vi "Logger.Variant.FindData4.vi"() -> ()   [LabVIEW 2016] (continued)
 "D:/Maszup/WABCO/SVN/LaserMarkingStation/SOFTWARE/logs/results1/old/170419233635 899 053 814 4.tdms", "Serials"=["480003047015824401617", "480003047015824411617", "480003047015824421617", "480003047015824431617", "480003047015824441617", "480003047015824451617", "480003047015824461617", "480003047015824471617", "480003047015824481617", "480003047015824491617", "480003047015824501617", "480003047015824511617", "480003047015824521617", "480003047015824531617", "480003047015824541617", "480003047015824551617", "480003047015824561617", "480003047015824571617", "480003047015824581617", "480003047015824591617", "480003047015824601617", "480003047015824611617", "480003047015824621617", "480003047015824631617", "480003047015824641617", "480003047015824651617", "480003047015824661617", "480003047015824671617", "480003047015824681617", "480003047015824691617", "480003047015824701617", "480003047015824711617", "480003047015824721617", "480003047015824731617", "480003047015824741617", "480003047015824751617", "480003047015824761617", "480003047015824771617", "480003047015824781617", "480003047015824791617"]}, {"Product"="9650010550", "Plate"="8990538144", "Path"=path "D:/Maszup/WABCO/SVN/LaserMarkingStation/SOFTWARE/logs/results1/old/170419234304 899 053 814 4.tdms", "Serials"=["965001055001223591617", "965001055001223601617", "965001055001223611617", "965001055001223621617", "965001055001223631617", "965001055001223641617", "965001055001223651617", "965001055001223661617", "965001055001223671617", "965001055001223681617", "965001055001223691617", "965001055001223701617"]}, {"Product"="9650010550", "Plate"="8990538144", "Path"=path "D:/Maszup/WABCO/SVN/LaserMarkingStation/SOFTWARE/logs/results1/old/170419234627 899 053 814 4.tdms", "Serials"=["965001055001223711617", "965001055001223721617", "965001055001223731617", "965001055001223741617", "965001055001223761617", "965001055001223771617", "965001055001223781617", "965001055001223791617", "965001055001223801617", "965001055001223811617", "965001055001223821617"]}, {"Product"="9650010550", "Plate"="8990538144", "Path"=path "D:/Maszup/WABCO/SVN/LaserMarkingStation/SOFTWARE/logs/results1/old/170419235443 899 053 814 4.tdms", "Serials"=["965001055001223711617", "965001055001223721617"]}, {"Product"="9650010550", "Plate"="8990538144", "Path"=path "D:/Maszup/WABCO/SVN/LaserMarkingStation/SOFTWARE/logs/results1/old/170420000204 899 053 814 4.tdms", "Serials"=["965001055001223711617", "965001055001223721617", "965001055001223731617", "965001055001223741617", "965001055001223751617", "965001055001223761617", "965001055001223771617", "965001055001223781617", "965001055001223791617", "965001055001223801617", "965001055001223811617", "965001055001223821617"]}, {"Product"="9650010550", "Plate"="8990538144", "Path"=path "D:/Maszup/WABCO/SVN/LaserMarkingStation/SOFTWARE/logs/results1/old/170420000541 899 053 814 4.tdms", "Serials"=["965001055001223831617", "965001055001223841617", "965001055001223851617", "965001055001223861617", "965001055001223871617", "965001055001223881617", "965001055001223891617", "965001055001223901617", "965001055001223911617", "965001055001223921617", "965001055001223931617", "965001055001223941617"]}, {"Product"="4728901130", "Plate"="8990501474", "Path"=path "D:/Maszup/WABCO/SVN/LaserMarkingStation/SOFTWARE/logs/results1/old/170420001243 899 050 147 4.tdms", "Serials"=["472890113015857521617", "472890113015857531617", "472890113015857541617", "472890113015857551617", "472890113015857561617", "472890113015857571617", "472890113015857581617", "472890113015857591617", "472890113015857601617", "472890113015857611617", "472890113015857621617"]}, {"Product"="4728901130", "Plate"="8990501474", "Path"=path "D:/Maszup/WABCO/SVN/LaserMarkingStation/SOFTWARE/logs/results1/old/170420001628 899 050 147 4.tdms", "Serials"=["472890113015857631617", "472890113015857641617", "472890113015857651617", "472890113015857661617", "472890113015857671617", "472890113015857681617"]}, {"Product"="4728901130", "Plate"="8990501474", "Path"=path "D:/Maszup/WABCO/SVN/LaserMarkingStation/SOFTWARE/logs/results1/old/170420002155 899 050 147 4.tdms", "Serials"=["472890113015857691617", "472890113015857701617", "472890113015857711617", "472890113015857721617", "472890113015857731617", "472890113015857741617", "472890113015857751617", "472890113015857761617", "472890113015857771617", "472890113015857781617", "472890113015857791617", "472890113015857801617", "472890113015857811617", "472890113015857821617", "472890113015857831617", "472890113015857841617", "472890113015857851617", "472890113015857861617", "472890113015857871617", "472890113015857881617", "472890113015857891617", "472890113015857901617", "472890113015857911617", "472890113015857921617", "472890113015857931617", "472890113015857941617", "472890113015857951617", "472890113015857961617", "472890113015857971617", "472890113015857981617", "472890113015857991617", "472890113015858001617", "472890113015858011617", "472890113015858021617", "472890113015858031617", "472890113015858041617"]}, {"Product"="9650010550", "Plate"="8990538144", "Path"=path "D:/Maszup/WABCO/SVN/LaserMarkingStation/SOFTWARE/logs/results1/old/170420002831 899 053 814 4.tdms", "Serials"=["965001055001223711617"]}, {"Product"="4728900500", "Plate"="8990538144", "Path"=path "D:/Maszup/WABCO/SVN/LaserMarkingStation/SOFTWARE/logs/results1/old/170420004617 899 053 814 4.tdms", "Serials"=["472890050016182201617", "472890050016182211617", "472890050016182221617", "472890050016182231617", "472890050016182241617", "472890050016182251617", "472890050016182261617", "472890050016182271617", "472890050016182281617", "472890050016182291617", "472890050016182301617", "472890050016182311617", "472890050016182321617", "472890050016182331617", "472890050016182341617", "472890050016182351617", "472890050016182361617", "472890050016182371617", "472890050016182381617", "472890050016182391617", "472890050016182401617", "472890050016182411617", "472890050016182421617", "472890050016182431617", "472890050016182441617", "472890050016182451617", "472890050016182461617", "472890050016182471617", "472890050016182481617", "472890050016182491617"]}, {"Product"="4728900500", "Plate"="8990538144", "Path"=path "D:/Maszup/WABCO/SVN/LaserMarkingStation/SOFTWARE/logs/results1/old/170420005019 899 053 814 4.tdms", "Serials"=["472890050016182501617", "472890050016182511617", "472890050016182521617", "472890050016182531617", "472890050016182541617", "472890050016182551617", "472890050016182561617", "472890050016182571617", "472890050016182581617", "472890050016182591617", "472890050016182601617", "472890050016182611617", "472890050016182621617", "472890050016182631617", "472890050016182641617", "472890050016182651617", "472890050016182661617", "472890050016182671617", "472890050016182681617", "472890050016182691617", "472890050016182701617", "472890050016182711617", "472890050016182721617", "472890050016182731617", "472890050016182741617", "472890050016182751617", "472890050016182761617", "472890050016182771617", "472890050016182781617", "472890050016182791617"]}, {"Product"="4728900500", "Plate"="8990538144", "Path"=path "D:/Maszup/WABCO/SVN/LaserMarkingStation/SOFTWARE/logs/results1/old/170420005540 899 053 814 4.tdms", "Serials"=["472890050016182801617", "472890050016182811617", "472890050016182821617", "472890050016182831617", "472890050016182841617", "472890050016182851617", "472890050016182861617", "472890050016182871617", "472890050016182881617"]}, {"Product"="4728900500", "Plate"="8990538144", "Path"=path "D:/Maszup/WABCO/SVN/LaserMarkingStation/SOFTWARE/logs/results1/old/170420010126 899 053 814 4.tdms", "Serials"=["472890050016182891617", "472890050016182901617", "472890050016182911617", "472890050016182921617", "472890050016182931617", "472890050016182941617", "472890050016182951617", "472890050016182961617", "472890050016182971617", "472890050016182981617", "472890050016182991617", "472890050016183001617", "472890050016183011617", "472890050016183021617", "472890050016183031617", "472890050016183041617", "472890050016183051617", "472890050016183061617", "472890050016183071617", "472890050016183081617", "472890050016183091617", "472890050016183101617", "472890050016183111617", "472890050016183121617", "472890050016183131617", "472890050016183141617", "472890050016183151617", "472890050016183161617", "472890050016183171617", "472890050016183181617"]}, {"Product"="4728900500", "Plate"="8990538144", "Path"=path "D:/Maszup/WABCO/SVN/LaserMarkingStation/SOFTWARE/logs/results1/old/170420010651 899 053 814 4.tdms", "Serials"=["472890050016183191617", "472890050016183201617", "472890050016183211617", "472890050016183221617", "472890050016183231617", "472890050016183241617", "472890050016183251617", "472890050016183261617", "472890050016183271617", "472890050016183281617", "472890050016183291617", "472890050016183301617", "472890050016183311617", "472890050016183321617", "472890050016183331617", "472890050016183341617", "472890050016183351617", "472890050016183361617", "472890050016183371617", "472890050016183381617", "472890050016183391617", "472890050016183401617", "472890050016183411617", "472890050016183421617", "472890050016183431617", "472890050016183441617", "472890050016183451617", "472890050016183461617", "472890050016183471617", "472890050016183481617"]}, {"Product"="4728901130", "Plate"="8990501474", "Path"=path "D:/Maszup/WABCO/SVN/LaserMarkingStation/SOFTWARE/logs/results1/old/170420011925 899 050 147 4.tdms", "Serials"=["472890113015858051617", "472890113015858061617", "472890113015858071617", "472890113015858081617", "472890113015858091617", "472890113015858101617", "472890113015858111617", "472890113015858121617", "472890113015858131617", "472890113015858141617", "472890113015858151617", "472890113015858161617", "472890113015858171617", "472890113015858181617", "472890113015858191617", "472890113015858201617", "472890113015858211617", "472890113015858221617", "472890113015858231617", "472890113015858241617", "472890113015858251617", "472890113015858261617", "472890113015858271617", "472890113015858281617", "472890113015858291617", "472890113015858301617", "472890113015858311617", "472890113015858321617", "472890113015858331617", "472890113015858341617", "472890113015858351617", "472890113015858361617", "472890113015858371617", "472890113015858381617", "472890113015858391617", "472890113015858401617"]}, {"Product"="4729051140", "Plate"="8990538154", "Path"=path "D:/Maszup/WABCO/SVN/LaserMarkingStation/SOFTWARE/logs/results1/old/170420013046 899 053 815 4.tdms", "Serials"=["472905114000051901617", "472905114000051911617"]}, {"Product"="9762001000", "Plate"="8990538144", "Path"=path "D:/Maszup/WABCO/SVN/LaserMarkingStation/SOFTWARE/logs/results1/old/170420020027 899 053 814 4.tdms", "Serials"=["976200100000055621617", "976200100000055631617"]}, {"Product"="9762001000", "Plate"="8990538144", "Path"=path "D:/Maszup/WABCO/SVN/LaserMarkingStation/SOFTWARE/logs/results1/old/170420020244 899 053 814 4.tdms", "Serials"=["976200100000055641617", "976200100000055651617"]}, {"Product"="9762001000", "Plate"="8990538144", "Path"=path "D:/Maszup/WABCO/SVN/LaserMarkingStation/SOFTWARE/logs/results1/old/170420020754 899 053 814 4.tdms", "Serials"=["976200100000055661617", "976200100000055671617"]}, {"Product"="9762001000", "Plate"="8990538144", "Path"=path "D:/Maszup/WABCO/SVN/LaserMarkingStation/SOFTWARE/logs/results1/old/170420030519 899 053 814 4.tdms", "Serials"=["976200100000055941617", "976200100000055951617", "976200100000055961617", "976200100000055971617", "976200100000055981617", "976200100000055991617", "976200100000056001617", "976200100000056011617", "976200100000056021617", "976200100000056031617", "976200100000056041617", "976200100000056051617", "976200100000056061617", "976200100000056071617", "976200100000056081617", "976200100000056091617", "976200100000056101617", "976200100000056111617", "976200100000056121617", "976200100000056131617", "976200100000056141617", "976200100000056151617", "976200100000056161617", "976200100000056171617", "976200100000056181617", "976200100000056191617", "976200100000056201617", "976200100000056211617", "976200100000056221617", "976200100000056231617", "976200100000056241617", "976200100000056251617", "976200100000056261617", "976200100000056271617", "976200100000056281617", "976200100000056291617", "976200100000056301617", "976200100000056311617", "976200100000056321617", "976200100000056331617", "976200100000056341617", "976200100000056351617", "976200100000056361617", "976200100000056371617", "976200100000056381617", "976200100000056391617", "976200100000056401617", "976200100000056411617", "976200100000056421617", "976200100000056431617", "976200100000056441617", "976200100000056451617", "976200100000056461617", "976200100000056471617", "976200100000056481617", "976200100000056491617", "976200100000056501617", "976200100000056511617", "976200100000056521617", "976200100000056531617", "976200100000056541617", "976200100000056551617", "976200100000056561617", "976200100000056571617", "976200100000056581617", "976200100000056591617", "976200100000056601617", "976200100000056611617", "976200100000056621617", "976200100000056631617", "976200100000056641617", "976200100000056651617", "976200100000056661617", "976200100000056671617", "976200100000056681617", "976200100000056691617", "976200100000056701617", "976200100000056711617", "976200100000056721617", "976200100000056731617", "976200100000056741617", "976200100000056751617", "976200100000056761617", "976200100000056771617", "976200100000056781617", "976200100000056791617", "976200100000056801617", "976200100000056811617", "976200100000056821617", "976200100000056831617", "976200100000056841617", "976200100000056851617", "976200100000056861617", "976200100000056871617", "976200100000056881617", "976200100000056891617", "976200100000056901617", "976200100000056911617", "976200100000056921617", "976200100000056931617", "976200100000056941617", "976200100000056951617", "976200100000056961617", "976200100000056971617"]}, {"Product"="4728900500", "Plate"="8990538144", "Path"=path "D:/Maszup/WABCO/SVN/LaserMarkingStation/SOFTWARE/logs/results1/old/170420034359 899 053 814 4.tdms", "Serials"=["472890050016183491617", "472890050016183501617", "472890050016183511617", "472890050016183521617", "472890050016183531617", "472890050016183541617", "472890050016183551617", "472890050016183561617", "472890050016183571617", "472890050016183581617", "472890050016183591617", "472890050016183601617", "472890050016183611617", "472890050016183621617", "472890050016183631617", "472890050016183641617", "472890050016183651617", "472890050016183661617", "472890050016183671617", "472890050016183681617", "472890050016183691617", "472890050016183701617", "472890050016183711617", "472890050016183721617", "472890050016183731617", "472890050016183741617", "472890050016183751617", "472890050016183761617", "472890050016183771617", "472890050016183781617"]}, {"Product"="4728900500", "Plate"="8990538144", "Path"=path "D:/Maszup/WABCO/SVN/LaserMarkingStation/SOFTWARE/logs/results1/old/170420034841 899 053 814 4.tdms", "Serials"=["472890050016183791617", "472890050016183801617", "472890050016183811617", "472890050016183821617", "472890050016183831617", "472890050016183841617", "472890050016183851617", "472890050016183861617", "472890050016183871617", "472890050016183881617", "472890050016183891617", "472890050016183901617", "472890050016183911617", "472890050016183921617", "472890050016183931617", "472890050016183941617", "472890050016183951617", "472890050016183961617", "472890050016183971617", "472890050016183981617", "472890050016183991617", "472890050016184001617", "472890050016184011617", "472890050016184021617", "472890050016184031617", "472890050016184041617", "472890050016184051617", "472890050016184061617", "472890050016184071617", "472890050016184081617"]}, {"Product"="4728800010", "Plate"="8990538154", "Path"=path "D:/Maszup/WABCO/SVN/LaserMarkingStation/SOFTWARE/logs/results1/old/170420042105 899 053 815 4.tdms", "Serials"=["472880001000599501617", "472880001000599511617", "472880001000599521617", "472880001000599531617", "472880001000599541617", "472880001000599551617"]}, {"Product"="4728800010", "Plate"="8990538154", "Path"=path "D:/Maszup/WABCO/SVN/LaserMarkingStation/SOFTWARE/logs/results1/old/170420042954 899 053 815 4.tdms", "Serials"=["472880001000599561617", "472880001000599571617", "472880001000599581617", "472880001000599591617", "472880001000599601617", "472880001000599611617"]}, {"Product"="9650010550", "Plate"="8990538144", "Path"=path "D:/Maszup/WABCO/SVN/LaserMarkingStation/SOFTWARE/logs/results1/old/170420164000 899 053 814 4.tdms", "Serials"=["965001055001224751617", "965001055001224761617", "965001055001224771617", "965001055001224781617"]}, {"Product"="9650010550", "Plate"="8990538144", "Path"=path "D:/Maszup/WABCO/SVN/LaserMarkingStation/SOFTWARE/logs/results1/old/170420171338 899 053 814 4.tdms", "Serials"=["965001055001224751617", "965001055001224761617", "965001055001224771617", "965001055001224781617"]}, {"Product"="9650010550", "Plate"="8990538144", "Path"=path "D:/Maszup/WABCO/SVN/LaserMarkingStation/SOFTWARE/logs/results1/old/170420172250 899 053 814 4.tdms", "Serials"=["965001055001224671617", "965001055001224681617", "965001055001224691617", "965001055001224701617", "965001055001224711617", "965001055001224721617"]}, {"Product"="4728800010", "Plate"="8990538154", "Path"=path "D:/Maszup/WABCO/SVN/LaserMarkingStation/SOFTWARE/logs/results1/old/170421085011 899 053 815 4.tdms", "Serials"=["472880001000599621617", "472880001000599631617", "472880001000599641617", "472880001000599651617"]}, {"Product"="4728800010", "Plate"="8990538154", "Path"=path "D:/Maszup/WABCO/SVN/LaserMarkingStation/SOFTWARE/logs/results1/old/170421085616 899 053 815 4.tdms", "Serials"=["472880001000599661617", "472880001000599671617"]}, {"Product"="9650010550", "Plate"="8990538144", "Path"=path "D:/Maszup/WABCO/SVN/LaserMarkingStation/SOFTWARE/logs/results2/new/170412140131 899 053 814 4.tdms", "Serials"=["965001055001217711517", "965001055001217721517", "965001055001217731517", "965001055001217741517", "965001055001217751517", "965001055001217761517", "965001055001217771517", "965001055001217781517", "965001055001217791517", "965001055001217801517", "965001055001217811517", "965001055001217821517"]}, {"Product"="9762001000", "Plate"="8990538144", "Path"=path "D:/Maszup/WABCO/SVN/LaserMarkingStation/SOFTWARE/logs/results2/new/170420090337 899 053 814 4.tdms", "Serials"=["976200100050002811617", "976200100050002821617", "976200100050002831617", "976200100050002841617"]}, {"Product"="9762001000", "Plate"="8990538144", "Path"=path "D:/Maszup/WABCO/SVN/LaserMarkingStation/SOFTWARE/logs/results2/new/170420090823 899 053 814 4.tdms", "Serials"=["976200100050002811617", "976200100050002821617", "976200100050002831617", "976200100050002841617", "976200100050002851617", "976200100050002861617", "976200100050002871617", "976200100050002881617", "976200100050002891617", "976200100050002901617", "976200100050002911617", "976200100050002921617", "976200100050002931617", "976200100050002941617", "976200100050002951617", "976200100050002961617", "976200100050002971617", "976200100050002981617", "976200100050002991617", "976200100050003001617", "976200100050003011617", "976200100050003021617", "976200100050003031617", "976200100050003041617", "976200100050003051617", "976200100050003061617", "976200100050003071617", "976200100050003081617", "976200100050003091617", "976200100050003101617", "976200100050003111617", "976200100050003121617", "976200100050003131617", "976200100050003141617", "976200100050003151617", "976200100050003161617", "976200100050003171617"]}, {"Product"="4800030470", "Plate"="8990538144", "Path"=path "D:/Maszup/WABCO/SVN/LaserMarkingStation/SOFTWARE/logs/results2/new/170420091613 899 053 814 4.tdms", "Serials"=["480003047053240011617", "480003047053240021617"]}, {"Product"="9650010550", "Plate"="8990538144", "Path"=path "D:/Maszup/WABCO/SVN/LaserMarkingStation/SOFTWARE/logs/results2/new/170420091916 899 053 814 4.tdms", "Serials"=["965001055001224061617"]}, {"Product"="4800030500", "Plate"="8990501474", "Path"=path "D:/Maszup/WABCO/SVN/LaserMarkingStation/SOFTWARE/logs/results2/new/170420092534 899 050 147 4.tdms", "Serials"=["480003050053240011617", "480003050053240021617", "480003050053240031617", "480003050053240041617", "480003050053240051617", "480003050053240061617", "480003050053240071617", "480003050053240081617", "480003050053240091617", "480003050053240101617", "480003050053240111617", "480003050053240121617", "480003050053240131617", "480003050053240141617", "480003050053240151617", "480003050053240161617", "480003050053240171617", "480003050053240181617", "480003050053240191617", "480003050053240201617", "480003050053240211617", "480003050053240221617", "480003050053240231617", "480003050053240241617", "480003050053240251617", "480003050053240261617", "480003050053240271617", "480003050053240281617", "480003050053240291617", "480003050053240301617", "480003050053240311617", "480003050053240321617", "480003050053240331617", "480003050053240341617", "480003050053240351617", "480003050053240361617", "480003050053240371617", "480003050053240381617", "480003050053240391617", "480003050053240401617", "480003050053240411617", "480003050053240421617", "480003050053240431617", "480003050053240441617", "480003050053240451617", "480003050053240461617", "480003050053240471617", "480003050053240481617", "480003050053240491617", "480003050053240501617", "480003050053240511617", "480003050053240521617", "480003050053240531617", "480003050053240541617", "480003050053240551617", "480003050053240561617", "480003050053240571617", "480003050053240581617", "480003050053240591617", "480003050053240601617", "480003050053240611617", "480003050053240621617", "480003050053240631617", "480003050053240641617", "480003050053240651617", "480003050053240661617", "480003050053240671617", "480003050053240681617", "480003050053240691617", "480003050053240701617", "480003050053240711617", "480003050053240721617", "480003050053240731617", "480003050053240741617", "480003050053240751617", "480003050053240761617", "480003050053240771617", "480003050053240781617", "480003050053240791617", "480003050053240801617", "480003050053240811617", "480003050053240821617", "480003050053240831617", "480003050053240841617", "480003050053240851617", "480003050053240861617", "480003050053240871617", "480003050053240881617", "480003050053240891617", "480003050053240901617", "480003050053240911617", "480003050053240921617", "480003050053240931617", "480003050053240941617", "480003050053240951617", "480003050053240961617", "480003050053240971617", "480003050053240981617", "480003050053240991617", "480003050053241001617", "480003050053241011617", "480003050053241021617", "480003050053241031617", "480003050053241041617", "480003050053241051617", "480003050053241061617", "480003050053241071617", "480003050053241081617", "480003050053241091617", "480003050053241101617", "480003050053241111617", "480003050053241121617", "480003050053241131617", "480003050053241141617", "480003050053241151617", "480003050053241161617", "480003050053241171617", "480003050053241181617", "480003050053241191617", "480003050053241201617", "480003050053241211617", "480003050053241221617", "480003050053241231617", "480003050053241241617", "480003050053241251617", "480003050053241261617", "480003050053241271617", "480003050053241281617"]}, {"Product"="4728900500", "Plate"="8990538144", "Path"=path "D:/Maszup/WABCO/SVN/LaserMarkingStation/SOFTWARE/logs/results2/new/170420093924 899 053 814 4.tdms", "Serials"=["472890050053240011617", "472890050053240021617", "472890050053240031617", "472890050053240041617", "472890050053240051617", "472890050053240061617", "472890050053240071617", "472890050053240081617", "472890050053240091617", "472890050053240101617", "472890050053240111617", "472890050053240121617", "472890050053240131617", "472890050053240141617", "472890050053240151617", "472890050053240161617", "472890050053240171617", "472890050053240181617", "472890050053240191617", "472890050053240201617", "472890050053240211617", "472890050053240221617", "472890050053240231617", "472890050053240241617", "472890050053240251617", "472890050053240261617", "472890050053240271617", "472890050053240281617", "472890050053240291617", "472890050053240301617"]}, {"Product"="4728900500", "Plate"="8990538144", "Path"=path "D:/Maszup/WABCO/SVN/LaserMarkingStation/SOFTWARE/logs/results2/new/170420094257 899 053 814 4.tdms", "Serials"=["472890050053240311617", "472890050053240321617", "472890050053240331617", "472890050053240341617", "472890050053240351617", "472890050053240361617", "472890050053240371617", "472890050053240381617", "472890050053240391617", "472890050053240401617", "472890050053240411617", "472890050053240421617", "472890050053240431617", "472890050053240441617", "472890050053240451617", "472890050053240461617", "472890050053240471617", "472890050053240481617", "472890050053240491617", "472890050053240501617", "472890050053240511617", "472890050053240521617", "472890050053240531617", "472890050053240541617", "472890050053240551617", "472890050053240561617", "472890050053240571617", "472890050053240581617", "472890050053240591617", "472890050053240601617"]}, {"Product"="4729051140", "Plate"="8990538154", "Path"=path "D:/Maszup/WABCO/SVN/LaserMarkingStation/SOFTWARE/logs/results2/new/170420094616 899 053 815 4.tdms", "Serials"=["472905114050026961617", "472905114050026971617", "472905114050026981617", "472905114050026991617", "472905114050027001617", "472905114050027011617", "472905114050027021617", "472905114050027031617", "472905114050027041617", "472905114050027051617", "472905114050027061617", "472905114050027071617", "472905114050027081617", "472905114050027091617", "472905114050027101617", "472905114050027111617", "472905114050027121617", "472905114050027131617", "472905114050027141617", "472905114050027151617", "472905114050027161617", "472905114050027171617", "472905114050027181617", "472905114050027191617", "472905114050027201617", "472905114050027211617", "472905114050027221617", "472905114050027231617", "472905114050027241617", "472905114050027251617", "472905114050027261617", "472905114050027271617", "472905114050027281617", "472905114050027291617", "472905114050027301617", "472905114050027311617", "472905114050027321617", "472905114050027331617", "472905114050027341617", "472905114050027351617", "472905114050027361617", "472905114050027371617", "472905114050027381617", "472905114050027391617", "472905114050027401617", "472905114050027411617", "472905114050027421617", "472905114050027431617", "472905114050027441617", "472905114050027451617", "472905114050027461617", "472905114050027471617", "472905114050027481617", "472905114050027491617", "472905114050027501617", "472905114050027511617", "472905114050027521617", "472905114050027531617", "472905114050027541617", "472905114050027551617", "472905114050027561617", "472905114050027571617", "472905114050027581617", "472905114050027591617", "472905114050027601617", "472905114050027611617", "472905114050027621617", "472905114050027631617", "472905114050027641617", "472905114050027651617", "472905114050027661617", "472905114050027671617"]}, {"Product"="4728901130", "Plate"="8990501474", "Path"=path "D:/Maszup/WABCO/SVN/LaserMarkingStation/SOFTWARE/logs/results2/new/170420095213 899 050 147 4.tdms", "Serials"=["472890113055000011617", "472890113055000021617", "472890113055000031617", "472890113055000041617", "472890113055000051617", "472890113055000061617", "472890113055000071617", "472890113055000081617", "472890113055000091617", "472890113055000101617", "472890113055000111617", "472890113055000121617", "472890113055000131617", "472890113055000141617", "472890113055000151617", "472890113055000161617", "472890113055000171617", "472890113055000181617", "472890113055000191617", "472890113055000201617", "472890113055000211617", "472890113055000221617", "472890113055000231617", "472890113055000241617", "472890113055000251617", "472890113055000261617", "472890113055000271617", "472890113055000281617", "472890113055000291617", "472890113055000301617", "472890113055000311617", "472890113055000321617", "472890113055000331617", "472890113055000341617", "472890113055000351617", "472890113055000361617", "472890113055000371617"]}, {"Product"="4728800610", "Plate"="8990538154", "Path"=path "D:/Maszup/WABCO/SVN/LaserMarkingStation/SOFTWARE/logs/results2/new/170420095710 899 053 815 4.tdms", "Serials"=["472880061053240011617", "472880061053240021617", "472880061053240031617", "472880061053240041617", "472880061053240051617", "472880061053240061617", "472880061053240071617", "472880061053240081617", "472880061053240091617", "472880061053240101617", "472880061053240111617", "472880061053240121617", "472880061053240131617", "472880061053240141617", "472880061053240151617", "472880061053240161617", "472880061053240171617", "472880061053240181617", "472880061053240191617", "472880061053240201617", "472880061053240211617", "472880061053240221617", "472880061053240231617", "472880061053240241617", "472880061053240251617", "472880061053240261617", "472880061053240271617", "472880061053240281617", "472880061053240291617", "472880061053240301617", "472880061053240311617", "472880061053240321617", "472880061053240331617", "472880061053240341617", "472880061053240351617", "472880061053240361617", "472880061053240371617", "472880061053240381617", "472880061053240391617", "472880061053240401617", "472880061053240411617", "472880061053240421617", "472880061053240431617", "472880061053240441617", "472880061053240451617", "472880061053240461617", "472880061053240471617", "472880061053240481617", "472880061053240491617", "472880061053240501617", "472880061053240511617", "472880061053240521617", "472880061053240531617", "472880061053240541617", "472880061053240551617", "472880061053240561617", "472880061053240571617", "472880061053240581617", "472880061053240591617", "472880061053240601617", "472880061053240611617", "472880061053240621617", "472880061053240631617", "472880061053240641617", "472880061053240651617", "472880061053240661617", "472880061053240671617", "472880061053240681617", "472880061053240691617", "472880061053240701617", "472880061053240711617", "472880061053240721617", "472880061053240731617", "472880061053240741617", "472880061053240751617", "472880061053240761617", "472880061053240771617", "472880061053240781617", "472880061053240791617", "472880061053240801617", "472880061053240811617", "472880061053240821617", "472880061053240831617", "472880061053240841617", "472880061053240851617", "472880061053240861617", "472880061053240871617", "472880061053240881617", "472880061053240891617", "472880061053240901617", "472880061053240911617", "472880061053240921617", "472880061053240931617", "472880061053240941617", "472880061053240951617", "472880061053240961617", "472880061053240971617", "472880061053240981617", "472880061053240991617", "472880061053241001617", "472880061053241011617", "472880061053241021617", "472880061053241031617", "472880061053241041617", "472880061053241051617", "472880061053241061617", "472880061053241071617", "472880061053241081617", "472880061053241091617", "472880061053241101617", "472880061053241111617", "472880061053241121617", "472880061053241131617", "472880061053241141617", "472880061053241151617", "472880061053241161617", "472880061053241171617", "472880061053241181617", "472880061053241191617", "472880061053241201617"]}, {"Product"="4728900500", "Plate"="8990538144", "Path"=path "D:/Maszup/WABCO/SVN/LaserMarkingStation/SOFTWARE/logs/results2/new/170420100805 899 053 814 4.tdms", "Serials"=["472890050053240611617", "472890050053240621617", "472890050053240631617", "472890050053240641617", "472890050053240651617", "472890050053240661617", "472890050053240671617", "472890050053240681617", "472890050053240691617", "472890050053240701617", "472890050053240711617", "472890050053240721617", "472890050053240731617", "472890050053240741617", "472890050053240751617", "472890050053240761617", "472890050053240771617", "472890050053240781617", "472890050053240791617", "472890050053240801617", "472890050053240811617", "472890050053240821617", "472890050053240831617", "472890050053240841617", "472890050053240851617", "472890050053240861617", "472890050053240871617", "472890050053240881617", "472890050053240891617", "472890050053240901617"]}, {"Product"="4802040310", "Plate"="8990538144", "Path"=path "D:/Maszup/WABCO/SVN/LaserMarkingStation/SOFTWARE/logs/results2/new/170420101129 899 053 814 4.tdms", "Serials"=["480204031053240011617", "480204031053240021617", "480204031053240031617", "480204031053240041617", "480204031053240051617", "480204031053240061617", "480204031053240071617", "480204031053240081617", "480204031053240091617", "480204031053240101617", "480204031053240111617", "480204031053240121617", "480204031053240131617", "480204031053240141617", "480204031053240151617", "480204031053240161617", "480204031053240171617", "480204031053240181617", "480204031053240191617", "480204031053240201617", "480204031053240211617", "480204031053240221617", "480204031053240231617", "480204031053240241617", "480204031053240251617", "480204031053240261617", "480204031053240271617", "480204031053240281617", "480204031053240291617", "480204031053240301617", "480204031053240311617", "480204031053240321617", "480204031053240331617", "480204031053240341617", "480204031053240351617", "480204031053240361617", "480204031053240371617", "480204031053240381617", "480204031053240391617", "480204031053240401617", "480204031053240411617", "480204031053240421617", "480204031053240431617", "480204031053240441617", "480204031053240451617"]}, {"Product"="9760001070", "Plate"="8990538144", "Path"=path "D:/Maszup/WABCO/SVN/LaserMarkingStation/SOFTWARE/logs/results2/new/170420101533 899 053 814 4.tdms", "Serials"=["976000107050001731617", "976000107050001741617", "976000107050001751617", "976000107050001761617", "976000107050001771617", "976000107050001781617", "976000107050001791617", "976000107050001801617", "976000107050001811617", "976000107050001821617", "976000107050001831617", "976000107050001841617", "976000107050001851617", "976000107050001861617", "976000107050001871617", "976000107050001881617", "976000107050001891617", "976000107050001901617", "976000107050001911617", "976000107050001921617", "976000107050001931617", "976000107050001941617", "976000107050001951617", "976000107050001961617", "976000107050001971617", "976000107050001981617", "976000107050001991617", "976000107050002001617", "976000107050002011617", "976000107050002021617", "976000107050002031617", "976000107050002041617", "976000107050002051617", "976000107050002061617", "976000107050002071617", "976000107050002081617", "976000107050002091617", "976000107050002101617", "976000107050002111617", "976000107050002121617", "976000107050002131617", "976000107050002141617", "976000107050002151617", "976000107050002161617", "976000107050002171617", "976000107050002181617", "976000107050002191617", "976000107050002201617", "976000107050002211617", "976000107050002221617", "976000107050002231617", "976000107050002241617", "976000107050002251617", "976000107050002261617", "976000107050002271617", "976000107050002281617", "976000107050002291617", "976000107050002301617", "976000107050002311617", "976000107050002321617", "976000107050002331617", "976000107050002341617", "976000107050002351617", "976000107050002361617", "976000107050002371617", "976000107050002381617", "976000107050002391617", "976000107050002401617", "976000107050002411617", "976000107050002421617", "976000107050002431617", "976000107050002441617", "976000107050002451617", "976000107050002461617", "976000107050002471617", "976000107050002481617", "976000107050002491617", "976000107050002501617", "976000107050002511617", "976000107050002521617", "976000107050002531617", "976000107050002541617", "976000107050002551617", "976000107050002561617", "976000107050002571617", "976000107050002581617", "976000107050002591617", "976000107050002601617", "976000107050002611617", "976000107050002621617", "976000107050002631617", "976000107050002641617", "976000107050002651617", "976000107050002661617", "976000107050002671617", "976000107050002681617", "976000107050002691617", "976000107050002701617", "976000107050002711617", "976000107050002721617", "976000107050002731617", "976000107050002741617", "976000107050002751617", "976000107050002761617", "976000107050002771617", "976000107050002781617", "976000107050002791617", "976000107050002801617", "976000107050002811617", "976000107050002821617", "976000107050002831617", "976000107050002841617", "976000107050002851617", "976000107050002861617", "976000107050002871617", "976000107050002881617", "976000107050002891617", "976000107050002901617", "976000107050002911617", "976000107050002921617", "976000107050002931617", "976000107050002941617", "976000107050002951617", "976000107050002961617", "976000107050002971617", "976000107050002981617", "976000107050002991617", "976000107050003001617", "976000107050003011617", "976000107050003021617", "976000107050003031617", "976000107050003041617", "976000107050003051617", "976000107050003061617", "976000107050003071617"]}, {"Product"="4613330000", "Plate"="8990501474", "Path"=path "D:/Maszup/WABCO/SVN/LaserMarkingStation/SOFTWARE/logs/results2/new/170420102740 899 050 147 4.tdms", "Serials"=["461333000050000021617", "461333000050000031617", "461333000050000041617", "461333000050000051617", "461333000050000061617", "461333000050000071617", "461333000050000081617", "461333000050000091617", "461333000050000101617", "461333000050000111617", "461333000050000121617", "461333000050000131617", "461333000050000141617", "461333000050000151617", "461333000050000161617", "461333000050000171617", "461333000050000181617", "461333000050000191617", "461333000050000201617", "461333000050000211617", "461333000050000221617", "461333000050000231617", "461333000050000241617", "461333000050000251617", "461333000050000261617", "461333000050000271617", "461333000050000281617", "461333000050000291617", "461333000050000301617", "461333000050000311617", "461333000050000321617", "461333000050000331617", "461333000050000341617", "461333000050000351617", "461333000050000361617", "461333000050000371617", "461333000050000381617", "461333000050000391617", "461333000050000401617", "461333000050000411617", "461333000050000421617", "461333000050000431617", "461333000050000441617", "461333000050000451617", "461333000050000461617", "461333000050000471617", "461333000050000481617", "461333000050000491617", "461333000050000501617", "461333000050000511617", "461333000050000521617", "461333000050000531617", "461333000050000541617", "461333000050000551617", "461333000050000561617", "461333000050000571617", "461333000050000581617", "461333000050000591617", "461333000050000601617", "461333000050000611617", "461333000050000621617", "461333000050000631617", "461333000050000641617", "461333000050000651617"]}, {"Product"="9650010550", "Plate"="8990538144", "Path"=path "D:/Maszup/WABCO/SVN/LaserMarkingStation/SOFTWARE/logs/results2/new/170420103535 899 053 814 4.tdms", "Serials"=["965001055001224071617", "965001055001224081617", "965001055001224091617", "965001055001224101617", "965001055001224111617", "965001055001224121617", "965001055001224131617", "965001055001224141617", "965001055001224151617", "965001055001224161617", "965001055001224171617", "965001055001224181617"]}, {"Product"="4728900800", "Plate"="8990538144", "Path"=path "D:/Maszup/WABCO/SVN/LaserMarkingStation/SOFTWARE/logs/results2/new/170420103745 899 053 814 4.tdms", "Serials"=["472890080050000111617", "472890080050000121617", "472890080050000131617", "472890080050000141617", "472890080050000151617", "472890080050000161617", "472890080050000171617", "472890080050000181617", "472890080050000191617", "472890080050000201617", "472890080050000211617", "472890080050000221617", "472890080050000231617", "472890080050000241617", "472890080050000251617", "472890080050000261617", "472890080050000271617", "472890080050000281617", "472890080050000291617", "472890080050000301617", "472890080050000311617", "472890080050000321617", "472890080050000331617", "472890080050000341617", "472890080050000351617", "472890080050000361617", "472890080050000371617", "472890080050000381617", "472890080050000391617", "472890080050000401617", "472890080050000411617", "472890080050000421617", "472890080050000431617", "472890080050000441617", "472890080050000451617", "472890080050000461617", "472890080050000471617", "472890080050000481617", "472890080050000491617", "472890080050000501617", "472890080050000511617", "472890080050000521617", "472890080050000531617", "472890080050000541617", "472890080050000551617", "472890080050000561617", "472890080050000571617", "472890080050000581617", "472890080050000591617", "472890080050000601617"]}, {"Product"="4728800610", "Plate"="8990538154", "Path"=path "D:/Maszup/WABCO/SVN/LaserMarkingStation/SOFTWARE/logs/results2/new/170420105254 899 053 815 4.tdms", "Serials"=["472880061053241211617", "472880061053241221617", "472880061053241231617", "472880061053241241617", "472880061053241251617", "472880061053241261617", "472880061053241271617", "472880061053241281617", "472880061053241291617", "472880061053241301617", "472880061053241311617", "472880061053241321617", "472880061053241331617", "472880061053241341617", "472880061053241351617", "472880061053241361617", "472880061053241371617", "472880061053241381617", "472880061053241391617", "472880061053241401617", "472880061053241411617", "472880061053241421617", "472880061053241431617", "472880061053241441617", "472880061053241451617", "472880061053241461617", "472880061053241471617", "472880061053241481617", "472880061053241491617", "472880061053241501617", "472880061053241511617", "472880061053241521617", "472880061053241531617", "472880061053241541617", "472880061053241551617", "472880061053241561617", "472880061053241571617", "472880061053241581617", "472880061053241591617", "472880061053241601617", "472880061053241611617", "472880061053241621617", "472880061053241631617", "472880061053241641617", "472880061053241651617", "472880061053241661617", "472880061053241671617", "472880061053241681617", "472880061053241691617", "472880061053241701617", "472880061053241711617", "472880061053241721617", "472880061053241731617", "472880061053241741617", "472880061053241751617", "472880061053241761617", "472880061053241771617", "472880061053241781617", "472880061053241791617", "472880061053241801617", "472880061053241811617", "472880061053241821617", "472880061053241831617", "472880061053241841617", "472880061053241851617", "472880061053241861617", "472880061053241871617", "472880061053241881617", "472880061053241891617", "472880061053241901617", "472880061053241911617", "472880061053241921617", "472880061053241931617", "472880061053241941617", "472880061053241951617", "472880061053241961617", "472880061053241971617", "472880061053241981617", "472880061053241991617", "472880061053242001617", "472880061053242011617", "472880061053242021617", "472880061053242031617", "472880061053242041617", "472880061053242051617", "472880061053242061617", "472880061053242071617", "472880061053242081617", "472880061053242091617", "472880061053242101617", "472880061053242111617", "472880061053242121617", "472880061053242131617", "472880061053242141617", "472880061053242151617", "472880061053242161617", "472880061053242171617", "472880061053242181617", "472880061053242191617", "472880061053242201617", "472880061053242211617", "472880061053242221617", "472880061053242231617", "472880061053242241617", "472880061053242251617", "472880061053242261617", "472880061053242271617", "472880061053242281617", "472880061053242291617", "472880061053242301617", "472880061053242311617", "472880061053242321617", "472880061053242331617", "472880061053242341617", "472880061053242351617", "472880061053242361617", "472880061053242371617", "472880061053242381617", "472880061053242391617", "472880061053242401617"]}, {"Product"="4640060000", "Plate"="8990538034", "Path"=path "D:/Maszup/WABCO/SVN/LaserMarkingStation/SOFTWARE/logs/results2/new/170420110948 899 053 803 4.tdms", "Serials"=["46400600000059201617", "46400600000059211617", "46400600000059221617", "46400600000059231617", "46400600000059241617", "46400600000059251617", "46400600000059261617", "46400600000059271617", "46400600000059281617", "46400600000059291617", "46400600000059301617", "46400600000059311617", "46400600000059321617", "46400600000059331617", "46400600000059341617", "46400600000059351617", "46400600000059361617", "46400600000059371617", "46400600000059381617", "46400600000059391617", "46400600000059401617", "46400600000059411617", "46400600000059421617", "46400600000059431617", "46400600000059441617", "46400600000059451617", "46400600000059461617", "46400600000059471617", "46400600000059481617", "46400600000059491617"]}, {"Product"="4801020600", "Plate"="8990538034", "Path"=path "D:/Maszup/WABCO/SVN/LaserMarkingStation/SOFTWARE/logs/results2/new/170420112103 899 053 803 4.tdms", "Serials"=["48010206001067311617"]}, {"Product"="4801020600", "Plate"="8990538034", "Path"=path "D:/Maszup/WABCO/SVN/LaserMarkingStation/SOFTWARE/logs/results2/new/170420112420 899 053 803 4.tdms", "Serials"=["48010206001067311617"]}, {"Product"="8840495050", "Plate"="8990538144", "Path"=path "D:/Maszup/WABCO/SVN/LaserMarkingStation/SOFTWARE/logs/results2/new/170420113720 899 053 814 4.tdms", "Serials"=["884049505000000161617", "884049505000000171617", "884049505000000181617", "884049505000000191617", "884049505000000201617", "884049505000000211617", "884049505000000221617", "884049505000000231617", "884049505000000241617", "884049505000000251617", "884049505000000261617", "884049505000000271617", "884049505000000281617", "884049505000000291617", "884049505000000301617", "884049505000000311617", "884049505000000321617", "884049505000000331617", "884049505000000341617", "884049505000000351617", "884049505000000361617", "884049505000000371617", "884049505000000381617", "884049505000000391617", "884049505000000401617", "884049505000000411617", "884049505000000421617", "884049505000000431617", "884049505000000441617", "884049505000000451617"]}, {"Product"="4728900500", "Plate"="8990538144", "Path"=path "D:/Maszup/WABCO/SVN/LaserMarkingStation/SOFTWARE/logs/results2/new/170420114337 899 053 814 4.tdms", "Serials"=["472890050053240911617", "472890050053240921617", "472890050053240931617", "472890050053240941617", "472890050053240951617", "472890050053240961617", "472890050053240971617", "472890050053240981617", "472890050053240991617", "472890050053241001617", "472890050053241011617", "472890050053241021617", "472890050053241031617", "472890050053241041617", "472890050053241051617", "472890050053241061617", "472890050053241071617", "472890050053241081617", "472890050053241091617", "472890050053241101617", "472890050053241111617", "472890050053241121617", "472890050053241131617", "472890050053241141617", "472890050053241151617", "472890050053241161617", "472890050053241171617", "472890050053241181617", "472890050053241191617", "472890050053241201617"]}, {"Product"="4801020350", "Plate"="8990538034", "Path"=path "D:/Maszup/WABCO/SVN/LaserMarkingStation/SOFTWARE/logs/results2/new/170420114836 899 053 803 4.tdms", "Serials"=["48010203501889871617", "48010203501889881617", "48010203501889891617", "48010203501889901617", "48010203501889911617", "48010203501889921617", "48010203501889931617", "48010203501889941617", "48010203501889951617", "48010203501889961617", "48010203501889971617", "48010203501889981617", "48010203501889991617", "48010203501890001617", "48010203501890011617", "48010203501890021617", "48010203501890031617", "48010203501890041617", "48010203501890051617", "48010203501890061617", "48010203501890071617", "48010203501890081617", "48010203501890091617", "48010203501890101617", "48010203501890111617", "48010203501890121617", "48010203501890131617", "48010203501890141617", "48010203501890151617", "48010203501890161617", "48010203501890171617", "48010203501890181617", "48010203501890191617", "48010203501890201617", "48010203501890211617", "48010203501890221617"]}, {"Product"="4801020800", "Plate"="8990538034", "Path"=path "D:/Maszup/WABCO/SVN/LaserMarkingStation/SOFTWARE/logs/results2/new/170420115209 899 053 803 4.tdms", "Serials"=["48010208000643611617", "48010208000643621617", "48010208000643631617", "48010208000643641617", "48010208000643651617", "48010208000643661617", "48010208000643671617", "48010208000643681617", "48010208000643691617", "48010208000643701617", "48010208000643711617", "48010208000643721617", "48010208000643731617", "48010208000643741617", "48010208000643751617", "48010208000643761617", "48010208000643771617", "48010208000643781617", "48010208000643791617", "48010208000643801617", "48010208000643811617", "48010208000643821617", "48010208000643831617", "48010208000643841617", "48010208000643851617", "48010208000643861617", "48010208000643871617", "48010208000643881617", "48010208000643891617", "48010208000643901617", "48010208000643911617", "48010208000643921617"]}, {"Product"="4801020800", "Plate"="8990538034", "Path"=path "D:/Maszup/WABCO/SVN/LaserMarkingStation/SOFTWARE/logs/results2/new/170420115554 899 053 803 4.tdms", "Serials"=["48010208000643211617", "48010208000643221617", "48010208000643231617", "48010208000643241617", "48010208000643251617", "48010208000643261617", "48010208000643271617", "48010208000643281617", "48010208000643291617", "48010208000643301617", "48010208000643311617", "48010208000643321617", "48010208000643331617", "48010208000643341617", "48010208000643351617", "48010208000643361617", "48010208000643371617", "48010208000643381617", "48010208000643391617", "48010208000643401617", "48010208000643411617", "48010208000643421617", "48010208000643431617", "48010208000643441617", "48010208000643451617", "48010208000643461617", "48010208000643471617", "48010208000643481617", "48010208000643491617", "48010208000643501617", "48010208000643511617", "48010208000643521617", "48010208000643531617", "48010208000643541617", "48010208000643551617", "48010208000643561617", "48010208000643571617", "48010208000643581617", "48010208000643591617", "48010208000643601617"]}, {"Product"="4640060000", "Plate"="8990538034", "Path"=path "D:/Maszup/WABCO/SVN/LaserMarkingStation/SOFTWARE/logs/results2/new/170420115932 899 053 803 4.tdms", "Serials"=["46400600000058601617", "46400600000058611617", "46400600000058621617", "46400600000058631617", "46400600000058641617", "46400600000058651617", "46400600000058661617", "46400600000058671617", "46400600000058681617", "46400600000058691617", "46400600000058701617", "46400600000058711617", "46400600000058721617", "46400600000058731617", "46400600000058741617", "46400600000058751617", "46400600000058761617", "46400600000058771617", "46400600000058781617", "46400600000058791617", "46400600000058801617", "46400600000058811617", "46400600000058821617", "46400600000058831617", "46400600000058841617", "46400600000058851617", "46400600000058861617", "46400600000058871617", "46400600000058881617", "46400600000058891617"]}, {"Product"="4728900500", "Plate"="8990538144", "Path"=path "D:/Maszup/WABCO/SVN/LaserMarkingStation/SOFTWARE/logs/results2/new/170420120606 899 053 814 4.tdms", "Serials"=["472890050053241211617", "472890050053241221617", "472890050053241231617", "472890050053241241617", "472890050053241251617", "472890050053241261617", "472890050053241271617", "472890050053241281617", "472890050053241291617", "472890050053241301617", "472890050053241311617", "472890050053241321617", "472890050053241331617", "472890050053241341617", "472890050053241351617", "472890050053241361617", "472890050053241371617", "472890050053241381617", "472890050053241391617", "472890050053241401617", "472890050053241411617", "472890050053241421617", "472890050053241431617", "472890050053241441617", "472890050053241451617", "472890050053241461617", "472890050053241471617", "472890050053241481617", "472890050053241491617", "472890050053241501617"]}, {"Product"="9650010550", "Plate"="8990538144", "Path"=path "D:/Maszup/WABCO/SVN/LaserMarkingStation/SOFTWARE/logs/results2/new/170420120954 899 053 814 4.tdms", "Serials"=["965001055001224311617", "965001055001224321617", "965001055001224331617", "965001055001224341617", "965001055001224351617", "965001055001224361617", "965001055001224371617", "965001055001224381617", "965001055001224391617", "965001055001224401617", "965001055001224411617", "965001055001224421617"]}, {"Product"="9650010550", "Plate"="8990538144", "Path"=path "D:/Maszup/WABCO/SVN/LaserMarkingStation/SOFTWARE/logs/results2/new/170420121134 899 053 814 4.tdms", "Serials"=["965001055001224191617", "965001055001224201617", "965001055001224211617", "965001055001224221617", "965001055001224231617", "965001055001224241617", "965001055001224251617", "965001055001224261617", "965001055001224271617", "965001055001224281617", "965001055001224291617", "965001055001224301617"]}, {"Product"="4728800640", "Plate"="8990538154", "Path"=path "D:/Maszup/WABCO/SVN/LaserMarkingStation/SOFTWARE/logs/results2/new/170420121803 899 053 815 4.tdms", "Serials"=["472880064053240011617", "472880064053240021617", "472880064053240031617", "472880064053240041617", "472880064053240051617", "472880064053240061617", "472880064053240071617", "472880064053240081617", "472880064053240091617", "472880064053240101617", "472880064053240111617", "472880064053240121617", "472880064053240131617", "472880064053240141617", "472880064053240151617", "472880064053240161617", "472880064053240171617", "472880064053240181617", "472880064053240191617", "472880064053240201617", "472880064053240211617", "472880064053240221617", "472880064053240231617", "472880064053240241617"]}, {"Product"="4728800640", "Plate"="8990538154", "Path"=path "D:/Maszup/WABCO/SVN/LaserMarkingStation/SOFTWARE/logs/results2/new/170420122043 899 053 815 4.tdms", "Serials"=["472880064053240251617", "472880064053240261617", "472880064053240271617", "472880064053240281617", "472880064053240291617", "472880064053240301617", "472880064053240311617", "472880064053240321617", "472880064053240331617", "472880064053240341617", "472880064053240351617", "472880064053240361617", "472880064053240371617", "472880064053240381617", "472880064053240391617", "472880064053240401617", "472880064053240411617", "472880064053240421617", "472880064053240431617", "472880064053240441617", "472880064053240451617", "472880064053240461617", "472880064053240471617", "472880064053240481617"]}, {"Product"="4728800640", "Plate"="8990538154", "Path"=path "D:/Maszup/WABCO/SVN/LaserMarkingStation/SOFTWARE/logs/results2/new/170420122344 899 053 815 4.tdms", "Serials"=["472880064053240491617", "472880064053240501617", "472880064053240511617", "472880064053240521617", "472880064053240531617", "472880064053240541617", "472880064053240551617", "472880064053240561617", "472880064053240571617", "472880064053240581617", "472880064053240591617", "472880064053240601617", "472880064053240611617", "472880064053240621617", "472880064053240631617", "472880064053240641617", "472880064053240651617", "472880064053240661617", "472880064053240671617", "472880064053240681617", "472880064053240691617", "472880064053240701617", "472880064053240711617", "472880064053240721617"]}, {"Product"="4802040310", "Plate"="8990538144", "Path"=path "D:/Maszup/WABCO/SVN/LaserMarkingStation/SOFTWARE/logs/results2/new/170420122729 899 053 814 4.tdms", "Serials"=["480204031053240461617", "480204031053240471617", "480204031053240481617", "480204031053240491617", "480204031053240501617", "480204031053240511617", "480204031053240521617", "480204031053240531617", "480204031053240541617", "480204031053240551617", "480204031053240561617", "480204031053240571617", "480204031053240581617", "480204031053240591617", "480204031053240601617", "480204031053240611617", "480204031053240621617", "480204031053240631617", "480204031053240641617", "480204031053240651617", "480204031053240661617", "480204031053240671617", "480204031053240681617", "480204031053240691617", "480204031053240701617", "480204031053240711617", "480204031053240721617", "480204031053240731617", "480204031053240741617", "480204031053240751617", "480204031053240761617", "480204031053240771617", "480204031053240781617", "480204031053240791617", "480204031053240801617", "480204031053240811617", "480204031053240821617", "480204031053240831617", "480204031053240841617", "480204031053240851617", "480204031053240861617", "480204031053240871617", "480204031053240881617", "480204031053240891617", "480204031053240901617"]}, {"Product"="4728900200", "Plate"="8990538144", "Path"=path "D:/Maszup/WABCO/SVN/LaserMarkingStation/SOFTWARE/logs/results2/new/170420123456 899 053 814 4.tdms", "Serials"=["472890020053240011617", "472890020053240021617", "472890020053240031617", "472890020053240041617", "472890020053240051617", "472890020053240061617", "472890020053240071617", "472890020053240081617", "472890020053240091617", "472890020053240101617", "472890020053240111617", "472890020053240121617", "472890020053240131617", "472890020053240141617", "472890020053240151617", "472890020053240161617", "472890020053240171617", "472890020053240181617", "472890020053240191617", "472890020053240201617", "472890020053240211617", "472890020053240221617", "472890020053240231617", "472890020053240241617", "472890020053240251617", "472890020053240261617", "472890020053240271617", "472890020053240281617", "472890020053240291617", "472890020053240301617"]}, {"Product"="4728900200", "Plate"="8990538144", "Path"=path "D:/Maszup/WABCO/SVN/LaserMarkingStation/SOFTWARE/logs/results2/new/170420123824 899 053 814 4.tdms", "Serials"=["472890020053240311617", "472890020053240321617", "472890020053240331617", "472890020053240341617", "472890020053240351617", "472890020053240361617", "472890020053240371617", "472890020053240381617", "472890020053240391617", "472890020053240401617", "472890020053240411617", "472890020053240421617", "472890020053240431617", "472890020053240441617", "472890020053240451617", "472890020053240461617", "472890020053240471617", "472890020053240481617", "472890020053240491617", "472890020053240501617", "472890020053240511617", "472890020053240521617", "472890020053240531617", "472890020053240541617", "472890020053240551617", "472890020053240561617", "472890020053240571617", "472890020053240581617", "472890020053240591617", "472890020053240601617"]}, {"Product"="4728900200", "Plate"="8990538144", "Path"=path "D:/Maszup/WABCO/SVN/LaserMarkingStation/SOFTWARE/logs/results2/new/170420124300 899 053 814 4.tdms", "Serials"=["472890020053240611617", "472890020053240621617", "472890020053240631617", "472890020053240641617", "472890020053240651617", "472890020053240661617", "472890020053240671617", "472890020053240681617", "472890020053240691617", "472890020053240701617", "472890020053240711617", "472890020053240721617", "472890020053240731617", "472890020053240741617", "472890020053240751617", "472890020053240761617", "472890020053240771617", "472890020053240781617", "472890020053240791617", "472890020053240801617", "472890020053240811617", "472890020053240821617", "472890020053240831617", "472890020053240841617", "472890020053240851617", "472890020053240861617", "472890020053240871617", "472890020053240881617", "472890020053240891617", "472890020053240901617"]}, {"Product"="9650010550", "Plate"="8990538144", "Path"=path "D:/Maszup/WABCO/SVN/LaserMarkingStation/SOFTWARE/logs/results2/new/170420124700 899 053 814 4.tdms", "Serials"=["965001055001224551617", "965001055001224561617", "965001055001224571617", "965001055001224581617", "965001055001224591617", "965001055001224601617", 
